vi "Ke2400 Config Multipoint.vi"(7 "Output Mode":u16(ring) items=["Fixed", "Sweep", "List"], 8 "error in (no error)":errorcluster, 9 "Trigger Count":i32, 10 "No of Time to Arm":i32, 11 "VISA resource name":refnum<visa-resource-name>) -> (0 "error out":errorcluster, 2 "resulting string":string, 3 "VISA resource name out":refnum<visa-resource-name>)   [LabVIEW 2012]
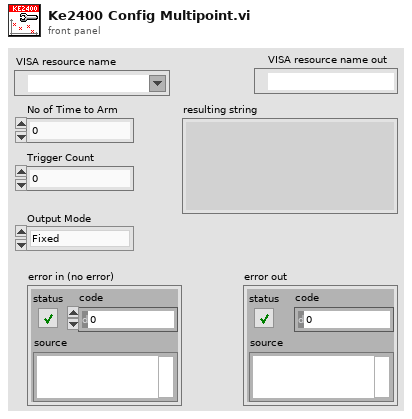
[diagram p1: front panel]
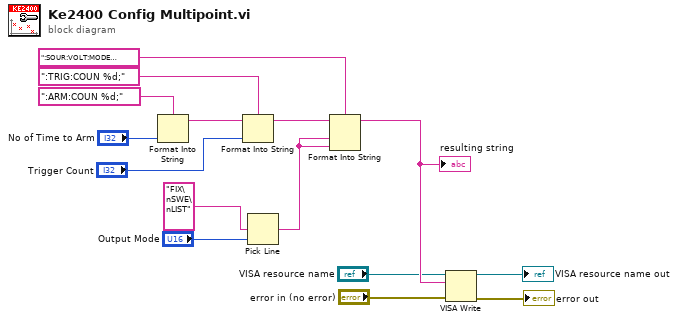
[diagram p0: block diagram]
diagram:
  n1 = Format Into String(format string=":ARM:COUN %d;", "No of Time to Arm") -> (resulting string=w14:string)  [unwired: 2 in, 1 out]
  n2 = Format Into String(format string=":TRIG:COUN %d;", initial string=w14, "Trigger Count") -> (resulting string=w12:string)  [unwired: 1 in, 1 out]
  n3 = Pick Line(multi-line string="FIX\nSWE\nLIST", line index="Output Mode") -> (output string=w8:string)  [unwired: 1 in]
  n4 = Format Into String(format string=":SOUR:VOLT:MODE %s;:SOUR:CURR:MODE %s;", initial string=w12, w8, w8) -> (resulting string=w7:string)  [unwired: 1 in, 1 out]
  "resulting string" <- w7
  n5 = VISA Write(VISA resource name="VISA resource name", write buffer=w7, error in (no error)="error in (no error)") -> (VISA resource name out=→"VISA resource name out":refnum<visa-resource-name>, error out=→"error out":errorcluster)  [unwired: 1 out]
